vi "VAttrbutes-Preview.vi"(6 "delimiter (/)":string="/", 8 "error in":errorcluster, 9 "ParentStr":string, 11 "VAttributes":variant) -> (0 "error out":errorcluster, 2 "Array":string[][](array[string]), 3 "VAttributes(dup)":variant)   [LabVIEW 2019]
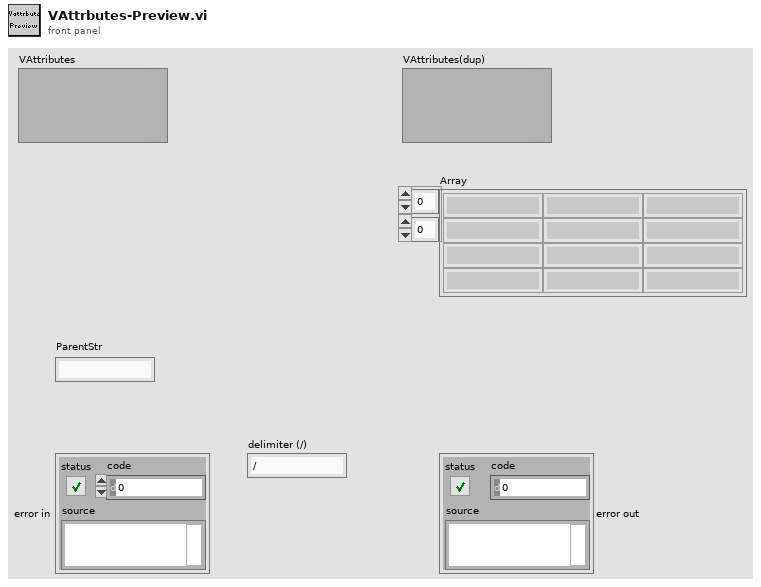
[diagram p1: front panel]
types:
  T1 = typedef "Type Descriptor Enumeration__ogtk.ctl" = enum8{"<Null>", "I8", "I16", "I32", "I64", "U8", "U16", "U32", "U64", "SGL", "DBL", "EXT", "CSG", "CDB", "CXT", "0x0F", "0x10", "0x11", "0x12", "0x13", "0x14", "Enum U8", "Enum U16", "Enum U32", "Enum U64", "SGL PQ", "DBL PQ", "EXT PQ", "CSG PQ", "CDB PQ", "CXT PQ", "0x1F", "0x20", "Boolean", "0x22", "0x23", "0x24", "0x25", "0x26", "0x27", "0x28", "0x29", "0x2A", "0x2B", "0x2C", "0x2D", "0x2E", "0x2F", "String", "0x31", "Path", "Pict", "0x34", "0x35", "0x36", "DAQ", "0x38", "0x39", "0x3A", "0x3B", "0x3C", "0x3D", "0x3E", "0x3F", "Array", "0x41", "0x42", "0x43", "0x44", "0x45", "0x46", "0x47", "0x48", "0x49", "0x4A", "0x4B", "0x4C", "0x4D", "0x4E", "0x4F", "Cluster", "0x51", "0x52", "Variant", "Waveform", "0x55", "0x56", "0x57", "0x58", "0x59", "0x5A", "0x5B", "0x5C", "0x5D", "0x5E", "0x5F", "0x60", "0x61", "0x62", "0x63", "0x64", "0x65", "0x66", "0x67", "0x68", "0x69", "0x6A", "0x6B", "0x6C", "0x6D", "0x6E", "0x6F", "Refnum"}
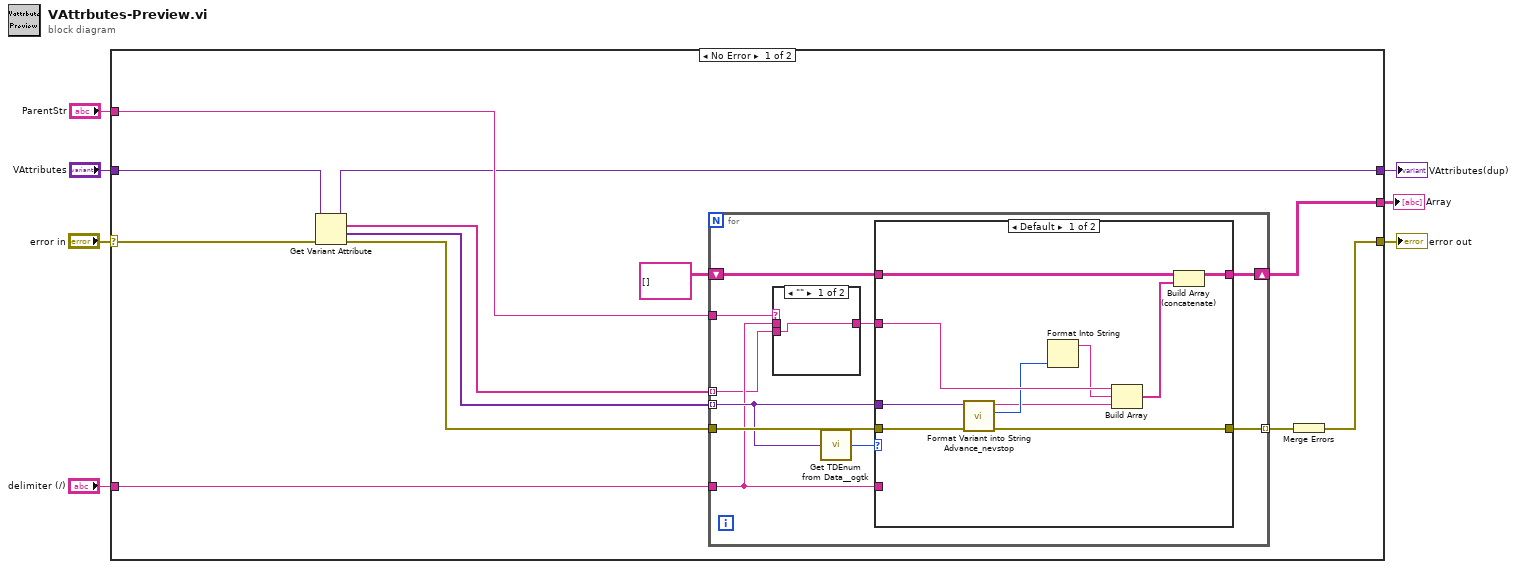
[diagram p0: block diagram]
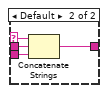
[diagram p2: hidden frame]
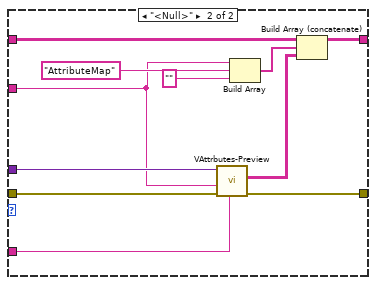
[diagram p3: hidden frame]
diagram:
  n1 = case shown="No Error" "error in" {
    selector: "error in" -> [w19 w57]
    tunnel: "VAttributes" -> [w10 w56]
    tunnel: [w9 w56] -> w5
    tunnel: [w12 w57] -> w4
    tunnel: [w16 _] -> w3
    tunnel: "ParentStr" -> [w15 _]
    tunnel: "delimiter (/)" -> [w11 _]
    frame No Error {
      n2 = Get Variant Attribute(Variant=w10, error in=w19) -> (duplicate Variant=w9:variant, names=w17:string[], values=w18:variant[], error out=w8:errorcluster)  [unwired: 2 in]
      n3 = for {
        tunnel: w18 -> [w24] mode=indexing
        tunnel: w17 -> [w21] mode=indexing
        tunnel: w15 -> [w23]
        shift-right: [w27] -> w16
        shift-left: string[][] [] -> [w28]
        tunnel: w8 -> [w26]
        tunnel: [w29] -> w14 mode=indexing
        tunnel: w11 -> [w22]
        n4 = case shown="\"\"" w23 {
          selector: w23 -> [_ w33]
          tunnel: w21 -> [w30 w34]
          tunnel: [w30 w32] -> w20
          tunnel: w22 -> [_ w31]
          frame "" {
          }
          frame Default {
            n5 = Concatenate Strings(w33, w31, w34) -> (w32:string)
          }
        }
        n6 = call <userlib>:"Get TDEnum from Data__ogtk.vi"("Data"=w24) -> ("Type Descriptor Enumeration"=w25:T1)  [unwired: 4 in]
        n7 = case shown="Default" w25 {
          tunnel: w24 -> [w39 w46]
          tunnel: w26 -> [w38 w49]
          tunnel: [w37 w48] -> w29
          tunnel: w20 -> [w41 w45]
          tunnel: [w43 w54] -> w27
          tunnel: w28 -> [w44 w55]
          tunnel: w22 -> [_ w50]
          frame Default {
            n8 = call <userlib>:"Format Variant into String Advance_nevstop.vi"("error in (no error)"=w38, "Variant"=w39) -> ("error out"=w37:errorcluster, "Type Descriptor Enumeration"=w36:T1, "Data"=w35:string)  [unwired: 7 in]
            n9 = Format Into String(w36) -> (resulting string=w40:string)  [unwired: 3 in, 1 out]
            n10 = Build Array(w41, w40, w35) -> (w42:string[])
            n11 = Build Array (concatenate)(w44, w42) -> (w43:string[][])
          }
          frame "<Null>" {
            n12 = call "VAttrbutes-Preview.vi"("delimiter (/)"=w50, "error in"=w49, "ParentStr"=w45, "VAttributes"=w46) -> ("error out"=w48:errorcluster, "Array"=w47:string[][])  [unwired: 5 in, 1 out]
            n13 = Build Array(w45, "AttributeMap" ("element"), "" ("element")) -> (w52:string[])
            n14 = Build Array (concatenate)(w55, w52, w47) -> (w54:string[][])
          }
        }
      }
      n15 = Merge Errors(w14) -> (w12:errorcluster)
    }
    frame Error {
    }
  }
  "error out" <- w4
  "VAttributes(dup)" <- w5
  "Array" <- w3
